vi "Write Cell Boolean.vi"(0 "Report Ref In":T1, 1 "Row Index":i32, 2 "Column Index":i32, 3 "error in (no error)":errorcluster, 4 "Value":bool) -> (5 "Report Ref Out":T1, 6 "error out":errorcluster)   [LabVIEW 2026, in "XCel Report Engine.lvlib"]
doc: "Writes a Boolean value to a cell in the active worksheet.\n\nThe cell is specified by zero-based row and column coordinates. Coordinate (0, 0) corresponds to cell A1.\n\nThe value is stored as a native Excel Boolean value. Writing the value replaces any existing cell value or formula while preserving the cell's existing formatting.\n\nThis VI is an instance of the polymorphic Write Cell.vi."
uses:
  XCel Report Engine.lvlib
  Controls/Report Ref.ctl
  C:/Users/m.santucci/Documents/ChatGPT/LV_REPORT_ENGINE/LV/DotNet/XCelReportEngine.dll
  DotNet/XCelReportEngine.dll
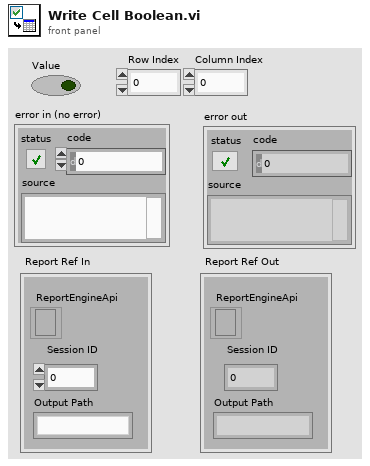
[diagram p1: front panel]
types:
  T1 = typedef "XCel Report Engine.lvlib/Report Ref.ctl" = cluster{"Session ID":i32, "Output Path":string, "ReportEngineApi":refnum<k24>}
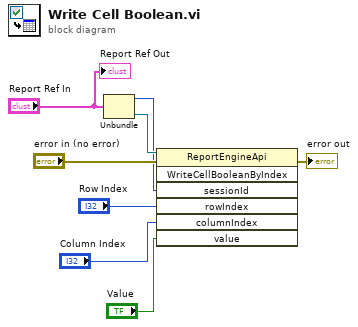
[diagram p0: block diagram]
diagram:
  n1 = Unbundle("Report Ref In") -> ("Session ID"=w4:i32, "ReportEngineApi"=w7:refnum<k24>)  [unwired: 1 out]
  n2 = invoke class="ReportEngineApi" method="WriteCellBooleanByIndex"(reference=w7, error in="error in (no error)", "sessionId"=w4, "rowIndex"="Row Index", "columnIndex"="Column Index", "value"="Value") -> (error out=→"error out":errorcluster)  [unwired: 1 in, 6 out]
  "Report Ref Out" <- "Report Ref In"
